vi "Initialize IDN.vi"(8 "error in (no error)":errorcluster, 11 "Instrument in":refnum<class "Instrument.lvclass">) -> (0 "error out":errorcluster, 3 "Instrument out":refnum<class "Instrument.lvclass">)   [LabVIEW 2019, in "Instrument.lvlib" / "Instrument.lvclass"]
doc: "Sets the <b>IDN</b> data field:\n- <b>vendor</b> is set by overriding <b>Get SMO Vendor.vi</b>\n- <b>model</b> is set by overriding <b>Get SMO Name.vi</b>\n- <b>serial</b> is set by overriding <b>Get SMO Serial Number.vi</b>\n- <b>firmware</b> refers to the version of your application"
uses:
  Instrument.lvclass
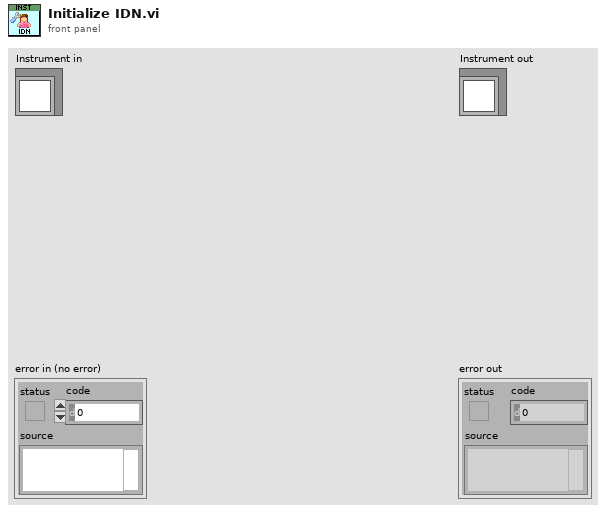
[diagram p1: front panel]
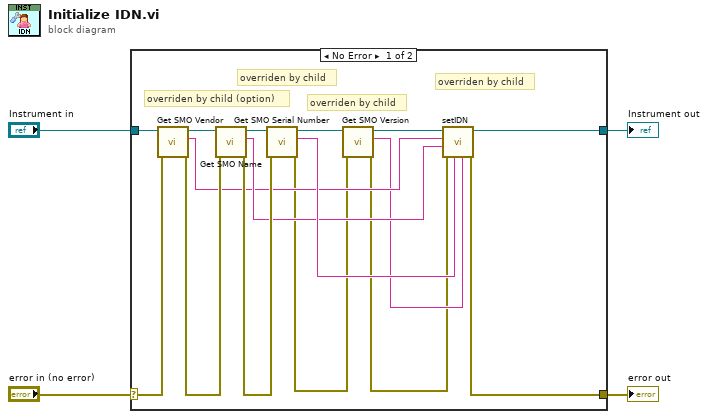
[diagram p0: block diagram]
diagram:
  n1 = case shown="No Error" "error in (no error)" {
    selector: "error in (no error)" -> [w16 w22]
    tunnel: [w13 w22] -> w3
    tunnel: [w19 w21] -> w1
    tunnel: "Instrument in" -> [w18 w21]
    frame No Error {
      # "overriden by child"
      # "overriden by child (option)"
      # "overriden by child"
      # "overriden by child"
      n2 = call-dynamic "Get SMO Vendor.vi"("error in (no error)"=w16, "Instrument in"=w18) -> ("error out"=w15:errorcluster, "SMO Vendor"=w10:string, "Instrument out"=w17:refnum<class "Instrument.lvclass">)  [unwired: 7 in]
      n3 = call-dynamic "Get SMO Name.vi"("error in (no error)"=w15, "Instrument in"=w17) -> ("error out"=w20:errorcluster, "SMO Name"=w11:string, "Instrument out"=w14:refnum<class "Instrument.lvclass">)  [unwired: 7 in]
      n4 = call-dynamic "Get SMO Serial Number.vi"("error in (no error)"=w20, "Instrument in"=w14) -> ("error out"=w6:errorcluster, "Serial Number"=w12:string, "Instrument out"=w9:refnum<class "Instrument.lvclass">)  [unwired: 7 in]
      n5 = call-dynamic "Get SMO Version.vi"("error in (no error)"=w6, "Instrument in"=w9) -> ("error out"=w5:errorcluster, "Version"=w7:string, "Instrument out"=w8:refnum<class "Instrument.lvclass">)  [unwired: 7 in]
      n6 = call "setIDN.vi"("Version"=w7, "Serial Number"=w12, "error in (no error)"=w5, "Name"=w11, "Vendor"=w10, "Instrument in"=w8) -> ("error out"=w13:errorcluster, "Instrument out"=w19:refnum<class "Instrument.lvclass">)  [unwired: 4 in]
    }
    frame Error {
    }
  }
  "error out" <- w3
  "Instrument out" <- w1
